vi "FROG_Wavelength2Omega.vi"(4 "Spectrum Info":T2, 5 "Experiment Trace":dbl[][](array[numeric])) -> (1 "Spectrum Info":T1, 2 "Converted Trace":dbl[][](array[numeric]))   [LabVIEW 2013]
uses:
  <vilib>/Analysis/6fits.llb/Curve Fitting Criteria.ctl
  <vilib>/Analysis/baseanly.llb/Quick Scale 2D.vi
  <vilib>/Analysis/NI_AALPro.lvlib
  <vilib>/gmath/NI_Gmath.lvlib
  <vilib>/Analysis/NI_AALBase.lvlib
panel:
  in  "Step Time":u16=100 format="%.0f ms"
  in  "Debug?":bool
  out "Interpolate Result":cluster{ext[], dbl[]}[](graph)
  out "Fitting":cluster{ext[], "Experiment Trace":dbl[]}[](graph)
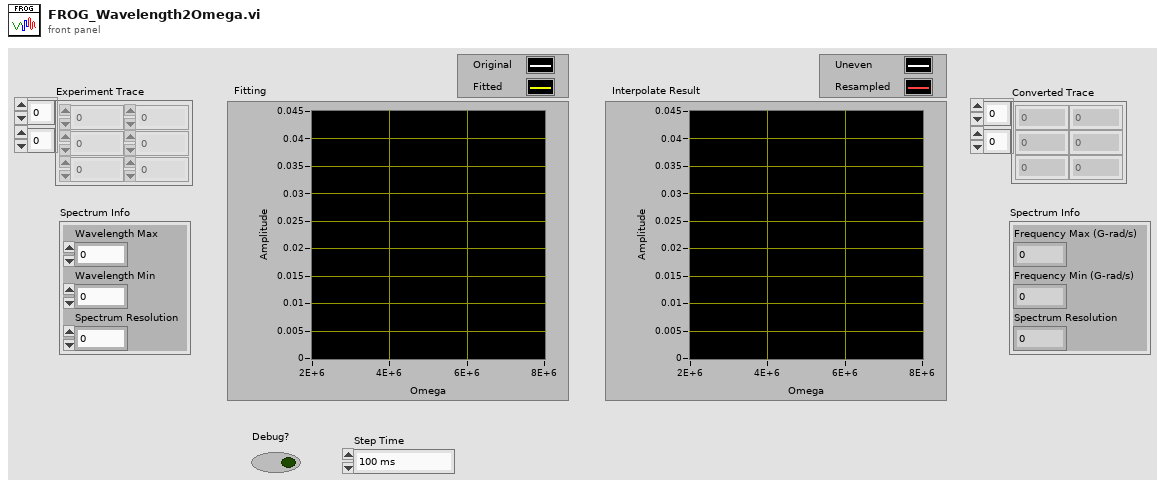
[diagram p1: front panel]
types:
  T1 = cluster{"Frequency Max (G-rad/s)":dbl, "Frequency Min (G-rad/s)":dbl, "Spectrum Resolution":u16}
  T2 = cluster{"Wavelength Max":dbl, "Wavelength Min":dbl, "Spectrum Resolution":u16}
  T3 = typedef "NI_AALPro.lvlib/Curve Fitting Criteria.ctl" = u16
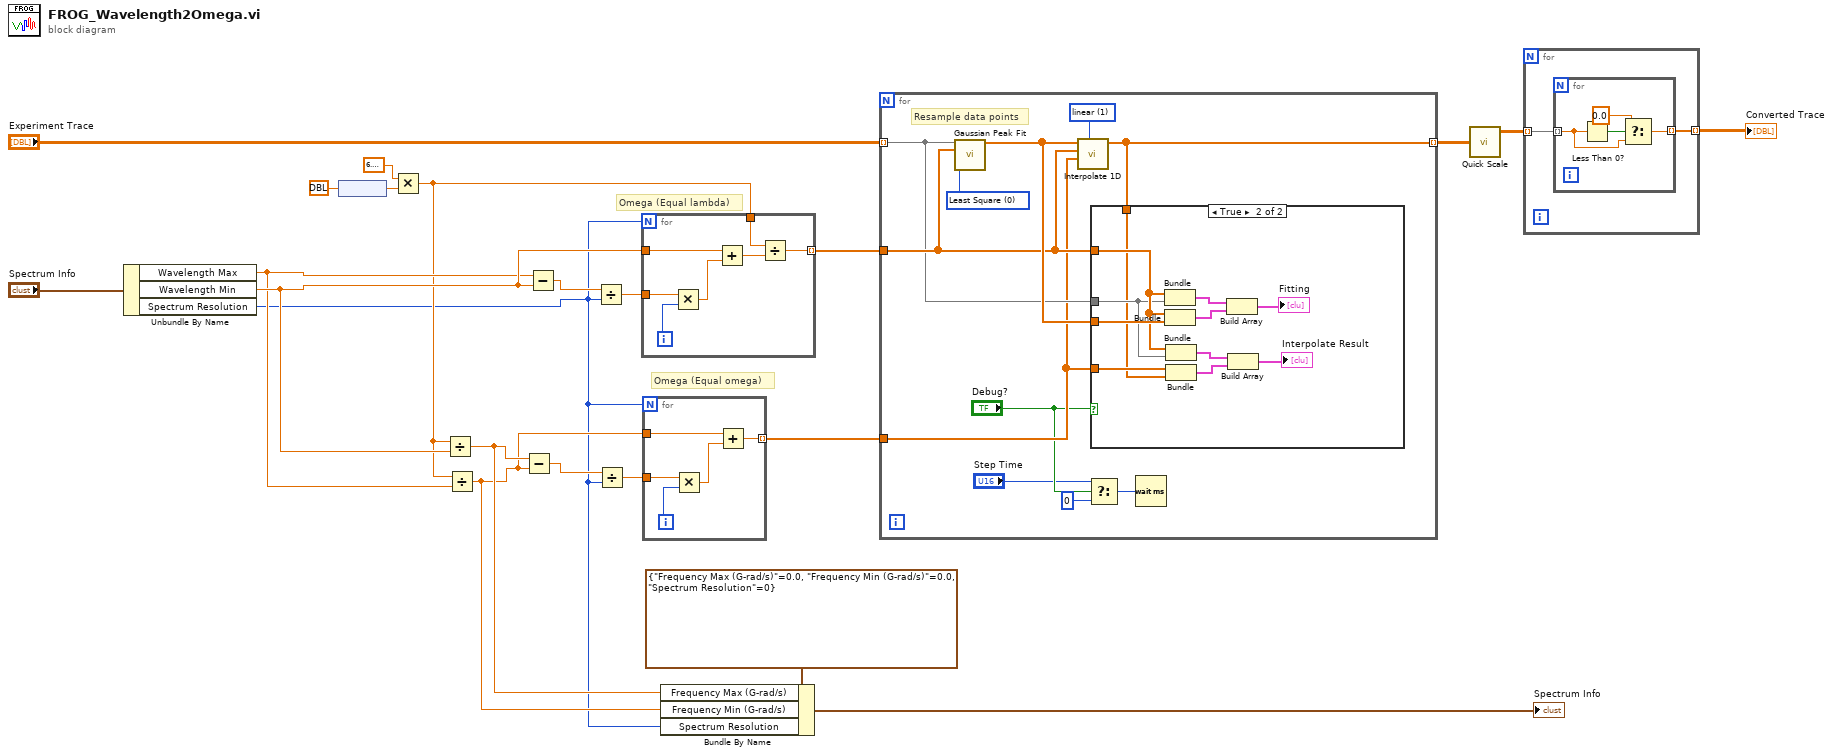
[diagram p0: block diagram]
diagram:
  # "Omega (Equal lambda)"
  # "Omega (Equal omega)"
  n1 = Unbundle By Name("Spectrum Info") -> ("Wavelength Max"=w10:dbl, "Wavelength Min"=w11:dbl, "Spectrum Resolution"=w4:u16)
  n2 = node(ext[unit] 299792458.0) -> (w17:ext)
  n3 = Multiply(x=6.283185307179586, y=w17) -> (x*y=w5:ext)
  n4 = Divide(x=w5, y=w11) -> (x/y=w8:ext)
  n5 = Divide(x=w5, y=w10) -> (x/y=w7:ext)
  n6 = Subtract(x=w8, y=w7) -> (x-y=w12:ext)
  n7 = Subtract(x=w10, y=w11) -> (x-y=w21:dbl)
  n8 = Divide(x=w21, y=w4) -> (x/y=w20:dbl)
  n9 = Divide(x=w12, y=w4) -> (x/y=w16:ext)
  n10 = for {
    N: w4 -> [_]
    tunnel: w20 -> [w29]
    tunnel: w11 -> [w26]
    tunnel: [w23] -> w15 mode=indexing
    tunnel: w5 -> [w24]
    i -> [w28]
    n11 = Multiply(x=w29, y=w28) -> (x*y=w27:dbl)
    n12 = Add(x=w26, y=w27) -> (x+y=w25:dbl)
    n13 = Divide(x=w24, y=w25) -> (x/y=w23:ext)
  }
  n14 = for {
    N: w4 -> [_]
    tunnel: w16 -> [w34]
    tunnel: [w31] -> w13 mode=indexing
    tunnel: w7 -> [w30]
    i -> [w33]
    n15 = Multiply(x=w34, y=w33) -> (x*y=w32:ext)
    n16 = Add(x=w30, y=w32) -> (x+y=w31:ext)
  }
  n17 = Bundle By Name(cluster=T1 {"Frequency Max (G-rad/s)"=0.0, "Frequency Min (G-rad/s)"=0.0, "Spectrum Resolution"=0}, "Frequency Max (G-rad/s)"=w8, "Frequency Min (G-rad/s)"=w7, "Spectrum Resolution"=w4) -> (→"Spectrum Info":T1)
  n18 = for {
    tunnel: w15 -> [w42]
    tunnel: "Experiment Trace" -> [w41] mode=indexing
    tunnel: w13 -> [w40]
    tunnel: [w39] -> w3 mode=indexing
    w44 = 1 items=["nearest", "linear", "spline", "cubic Hermite", "Lagrange"] ("method")
    w45 = T3 0 items=["Least Square", "Least Absolute Residual", "Bisquare"] ("method")
    # "Resample data points"
    n19 = call <vilib>:"Gaussian Peak Fit.vi"("Y"=w41, "X"=w42, "method"=w45) -> ("Best Gaussian Fit"=w43:dbl[])  [unwired: 6 in, 6 out]
    n20 = call <vilib>:"Interpolate 1D.vi"("method"=w44, "xi"=w40, "X"=w42, "Y"=w43) -> ("yi"=w39:dbl[])  [unwired: 5 in, 2 out]
    n21 = Select(t="Step Time", s="Debug?", f=u16 0) -> (s? t:f=w35:u16)
    n22 = case shown="True" "Debug?" {
      tunnel: w43 -> [_ w53]
      tunnel: w42 -> [_ w50]
      tunnel: w41 -> [_ w49]
      tunnel: w40 -> [_ w48]
      tunnel: w39 -> [_ w47]
      frame False {
      }
      frame True {
        n23 = Bundle(w50, "Experiment Trace"=w49) -> (w56:cluster{ext[], "Experiment Trace":dbl[]})  [unwired: 1 in]
        n24 = Bundle(w50, "Best Gaussian Fit"=w53) -> (w55:cluster{ext[], "Best Gaussian Fit":dbl[]})  [unwired: 1 in]
        n25 = Bundle(w50, "Experiment Trace"=w49) -> (w52:cluster{ext[], "Experiment Trace":dbl[]})  [unwired: 1 in]
        n26 = Bundle(w48, "yi"=w47) -> (w51:cluster{ext[], "yi":dbl[]})  [unwired: 1 in]
        n27 = Build Array(w56, w55) -> (→"Fitting":cluster{ext[], "Best Gaussian Fit":dbl[]}[])
        n28 = Build Array(w52, w51) -> (→"Interpolate Result":cluster{ext[], "yi":dbl[]}[])
      }
    }
    n29 = Wait (ms)(milliseconds to wait=w35) -> ()  [unwired: 1 out]
  }
  n30 = call-poly <vilib>:"Quick Scale.vi"("X"=w3) -> ("Yij=Xij/Max|X|"=w2:dbl[][])  [unwired: 2 out]
  n31 = for {
    tunnel: w2 -> [w58] mode=indexing
    tunnel: [w57] -> w1 mode=indexing
    n32 = for {
      tunnel: w58 -> [w61] mode=indexing
      tunnel: [w59] -> w57 mode=indexing
      n33 = Less Than 0?(x=w61) -> (x < 0?=w62:bool)
      n34 = Select(t=0.0, s=w62, f=w61) -> (s? t:f=w59:dbl)
    }
  }
  "Converted Trace" <- w1
